vi "Write Header Data to file.vi"(8 "error in":errorcluster, 11 "Report Generator in":refnum<class "Report Generator.lvclass">) -> (0 "error out":errorcluster, 3 "Report Generator out":refnum<class "Report Generator.lvclass">)   [LabVIEW 2018, in "Report Generator.lvlib" / "Report Generator.lvclass"]
uses:
  Report Generator.lvclass
  Report Generator.lvclass/Report Generator.ctl
  <vilib>/Utility/file.llb/Write Delimited Spreadsheet (string).vi
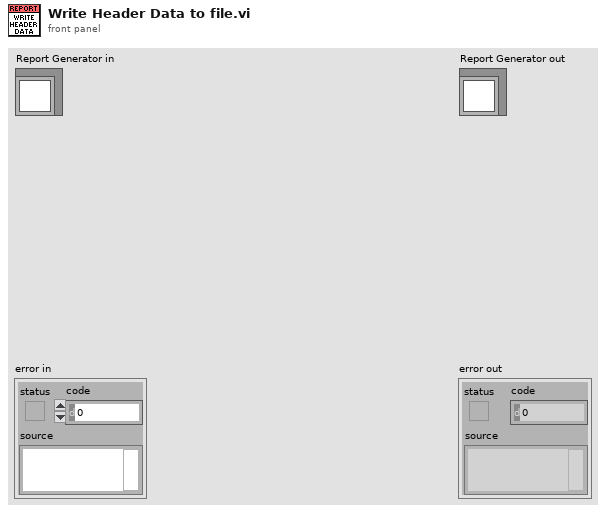
[diagram p1: front panel]
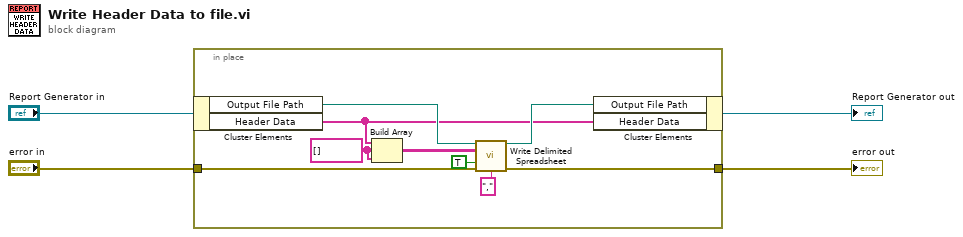
[diagram p0: block diagram]
diagram:
  n1 = in-place {
    in-place-border: [w10] -> w2
    in-place-border: "error in" -> [w8]
    w5 = string[] [] ("element")
    n2 = in-place-cluster #1("Report Generator in") -> ("Output File Path"=w13:path, "Header Data"=w7:string[])
    n3 = Build Array(w7, w5, w5) -> (w6:string[][])
    n4 = call-poly <vilib>:"Write Delimited Spreadsheet.vi"("file path (dialog if empty)"=w13, "2D data"=w6, "append to file? (new file:F)"=TRUE, "error in (no error)"=w8, "delimiter (\\t)"="," ("delimiter (\\t)")) -> ("new file path (Not A Path if cancelled)"=w12:path, "error out"=w10:errorcluster)  [unwired: 9 in]
    n5 = in-place-cluster #1("Output File Path"=w12, "Header Data"=w7) -> (→"Report Generator out":refnum<class "Report Generator.lvclass">)
  }
  "error out" <- w2
